vi "To Serial Form.vi"(6 "Serial Version":T1, 10 "Serializer in":refnum<class "Serializer.lvclass">, 11 "Switch in":refnum<class "Switch.lvclass">) -> (0 "error out":errorcluster, 2 "Serializer out":refnum<class "Serializer.lvclass">, 3 "Switch out":refnum<class "Switch.lvclass">)   [LabVIEW 2012]
uses:
  <userlib>/Serialization/Serializable/Serializable.lvclass
  <userlib>/Serialization/Serializable/Insert Double.vi
  <userlib>/Serialization/Serializable/Insert Boolean.vi
  <userlib>/Serialization/Serializer/Serializer.lvclass
  <userlib>/Serialization/Serialization Common/Serial Version.ctl
  <userlib>/Serialization/Serialization Common/Serialization Common.lvlib
  Switch.lvclass
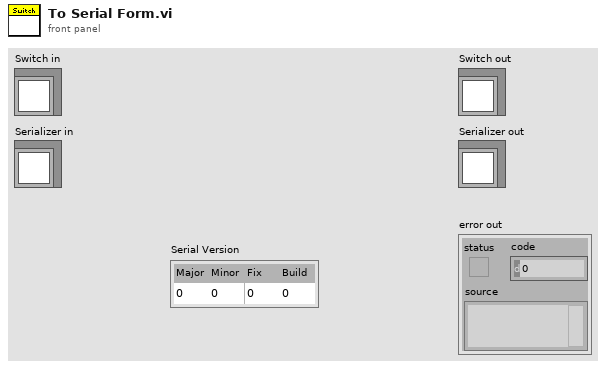
[diagram p1: front panel]
types:
  T1 = typedef "Serialization Common.lvlib/Serial Version.ctl" = cluster{"Major":u16, "Minor":u16, "Fix":u16, "Build":u16}
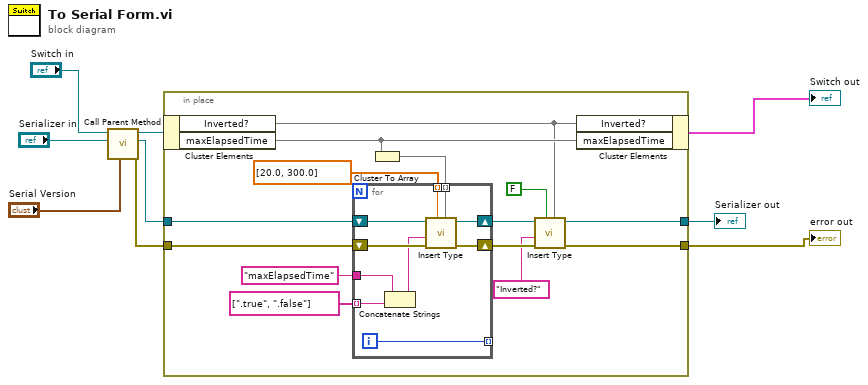
[diagram p0: block diagram]
diagram:
  n1 = call-parent "Call Parent Method"("Serial Version"="Serial Version", "Serializer in"="Serializer in", "Serializable in"="Switch in") -> ("error out"=w4:errorcluster, "Serializer out"=w5:refnum<class "Serializer.lvclass">, "Serializable out"=w6:refnum<class "Serializable.lvclass">)  [unwired: 6 in]
  n2 = in-place {
    in-place-border: w5 -> [w21]
    in-place-border: w4 -> [w16]
    in-place-border: [w12] -> w3
    in-place-border: [w11] -> w1
    n3 = in-place-cluster #1(w6) -> ("Inverted?"=w10, "maxElapsedTime"=w13)
    n4 = Cluster To Array(cluster=w13) -> (array=w20:void[])
    n5 = for {
      tunnel: string[] [".true", ".false"] -> [w33] mode=indexing
      tunnel: "maxElapsedTime" ("string") -> [w32]
      tunnel: w20 -> [w30] mode=indexing
      tunnel: dbl[] [20.0, 300.0] -> [w29] mode=indexing
      shift-right: [w27] -> w15
      shift-left: w16 -> [w26]
      tunnel: [w24] -> _ mode=indexing
      shift-right: [w28] -> w18
      shift-left: w21 -> [w31]
      i -> [w24]
      n6 = Concatenate Strings(w32, w33) -> (w25:string)
      n7 = call-poly <userlib>:"Insert Type.vi"("Double"=w30, "Default Value"=w29, "error in (no error)"=w26, "Name"=w25, "Serializer in"=w31) -> ("error out"=w27:errorcluster, "Serializer out"=w28:refnum<class "Serializer.lvclass">)  [unwired: 5 in]
    }
    n8 = call-poly <userlib>:"Insert Type.vi"("Boolean"=w10, "Default Value"=FALSE, "error in (no error)"=w15, "Name"="Inverted?", "Serializer in"=w18) -> ("error out"=w11:errorcluster, "Serializer out"=w12:refnum<class "Serializer.lvclass">)  [unwired: 5 in]
    n9 = in-place-cluster #1("Inverted?"=w10, "maxElapsedTime"=w13) -> (→"Switch out":cluster{})
  }
  "error out" <- w1
  "Serializer out" <- w3
